vi "Update Slot Display.vi"(8 "error in":errorcluster, 9 "Location":cluster{"X":i32, "Y":i32}, 10 "Button":i32, 11 "UI Actor in":refnum<class "UI Actor.lvclass">) -> (0 "error out":errorcluster, 3 "UI Actor out":refnum<class "UI Actor.lvclass">)   [LabVIEW 2024, in "UI Actor.lvlib" / "UI Actor.lvclass"]
uses:
  UI Actor.lvclass
  UI Actor.lvclass/UI Actor.ctl
  Controls/Communication Parameters.ctl
  <vilib>/JDP Science/JSONtext/Next JSON Value.vi
  <vilib>/JDP Science/JSONtext/String Subset.vi
  <vilib>/JDP Science/JSONtext/Parsing/Advance past next JSON Value (inlined COPY).vi
  <vilib>/JDP Science/JSONtext/Parsing/Advance past whitespace.vi
  <vilib>/JDP Science/JSONtext/Parsing/Advance past String.vi
  <vilib>/JDP Science/JSONtext/Parsing/Advance past Number.vi
  <vilib>/JDP Science/JSONtext/Parsing/Advance past Line Ending.vi
  PDO Grid/PDO Grid.lvclass
  D:/git/Sourcegrid-LabVIEW/source/Grid/SourceGrid.lvclass
  <vilib>/JDP Science/JSONtext/Parsing/Parse Full Path or Item Name.vi
  <vilib>/JDP Science/JSONtext/Parsing/Advance past Array.vi
  <vilib>/JDP Science/JSONtext/Parsing/Advance past Object.vi
  <vilib>/JDP Science/JSONtext/support/Error Cluster From Code.vi
  <vilib>/JDP Science/JSONtext/Offset/Find Item Locations by Path.vi
  Sourcegrid-LabVIEW/source/Cells/Cell/Cell.lvclass
  Sourcegrid-LabVIEW/source/Grid/SourceGrid.lvclass
  <vilib>/JDP Science/JSONtext/JSONtext.lvlib
panel:
  out "Transmission Type":u8(ring)=254 items=["synchronous (acyclic)"=0, "synchronous (cyclic every sync)"=1, "synchronous (cyclic every 2nd SYNC)"=2, "synchronous (cyclic every 3rd SYNC)"=3, "synchronous (cyclic every 4th SYNC)"=4, "synchronous (cyclic every 240th SYNC)"=240, "reserved"=241, "reserved"=251, "RTR-only (synchronous)"=252, "RTR-only (event-driven)"=253, "event-driven (manufacturer-specific)"=254, "event-driven (device profile and application profile specific)"=255]
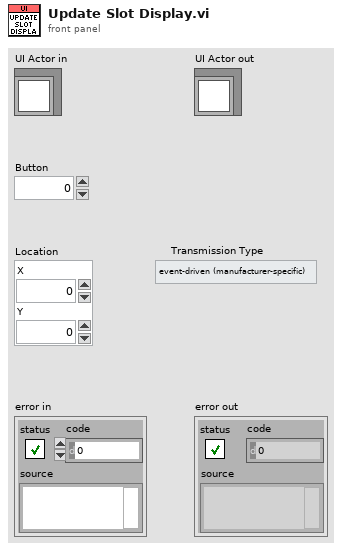
[diagram p1: front panel]
types:
  T1 = typedef "Communication Parameters.ctl" = cluster{"Communication":string, "Mapping":string, "COB":string, "Type":string, "Inhibit":string, "Event Timer":string, "Sync Start":string}
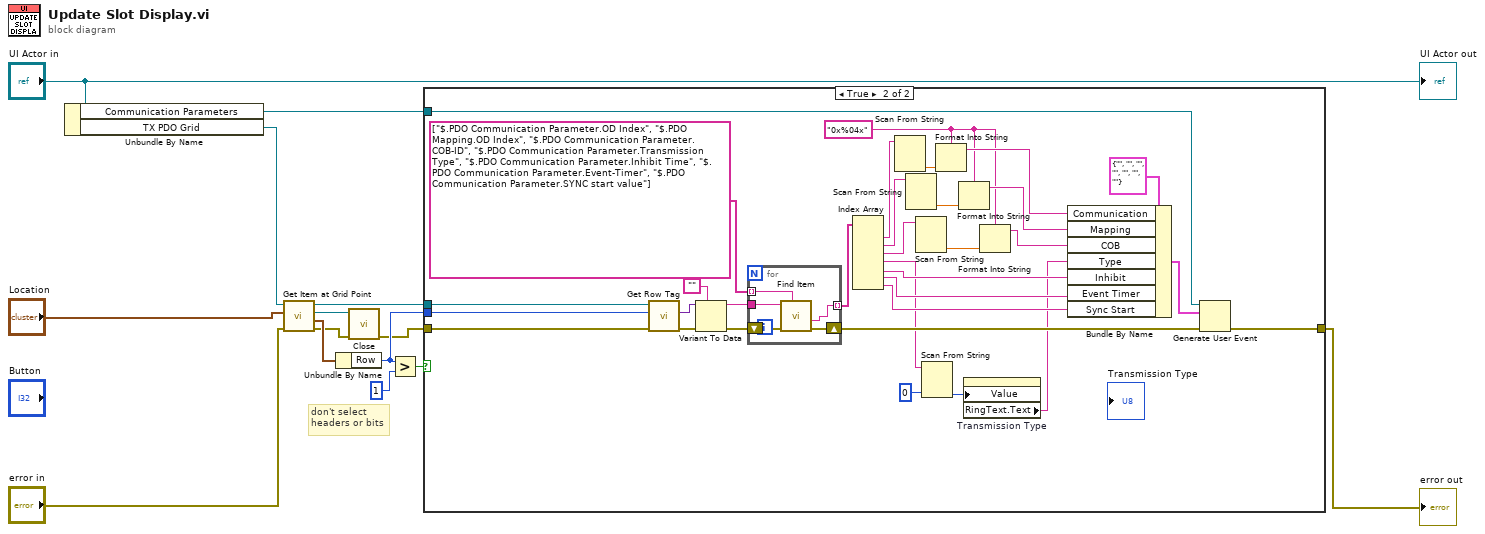
[diagram p0: block diagram]
diagram:
  # "don't select\nheaders or bits"
  n1 = Unbundle By Name("UI Actor in") -> ("Communication Parameters"=w1:refnum<user-event>, "TX PDO Grid"=w13:refnum<class "PDO Grid.lvclass">)
  n2 = call "Get Item at Grid Point.vi"("error in"="error in", "Location"="Location", "SourceGrid in"=w13) -> ("error out"=w8:errorcluster, "Cell Position"=w10:cluster{"Row":i32, "Column":i32}, "Cell out"=w2:refnum<class "Cell.lvclass">, "SourceGrid out"=w7:refnum<class "PDO Grid.lvclass">)  [unwired: 5 in]
  n3 = Unbundle By Name(w10) -> ("Row"=w5:i32)
  n4 = call-dynamic "Close.vi"("error in"=w8, "Cell in"=w2) -> ("error out"=w3:errorcluster)  [unwired: 8 in, 1 out]
  n5 = Greater?(x=w5, y=1) -> (0:w4:bool)
  n6 = case shown="True" w4 {
    tunnel: w3 -> [w15 w47]
    tunnel: w7 -> [_ w46]
    tunnel: [w15 w37] -> w6
    tunnel: w5 -> [_ w44]
    tunnel: w1 -> [_ w36]
    frame False {
    }
    frame True {
      w27 = "0x%04x" ("format string")
      n7 = call "Get Row Tag.vi"("error in"=w47, "Row Index"=w44, "SourceGrid in"=w46) -> ("error out"=w45:errorcluster, "object"=w43:variant)  [unwired: 6 in, 1 out]
      n8 = Variant To Data(error in=w45, type="", Variant=w43) -> (data=w41:string, error out=w39:errorcluster)
      n9 = for {
        tunnel: w41 -> [w49]
        tunnel: string[] ["$.PDO Communication Parameter.OD Index", "$.PDO Mapping.OD Index", "$.PDO Communication Parameter.COB-ID", "$.PDO Communication Parameter.Transmission Type", "$.PDO Communication Parameter.Inhibit Time", "$.PDO Communication Parameter.Event-Timer", "$.PDO Communication Parameter.SYNC start value"] -> [w52] mode=indexing
        shift-right: [w50] -> w38
        shift-left: w39 -> [w51]
        tunnel: [w48] -> w33 mode=indexing
        n10 = call <vilib>:"Find Item.vi"("$Path or Item Name"=w52, "error in (no error)"=w51, "JSON"=w49) -> ("error out"=w50:errorcluster, "<JSON>"=w48:string)  [unwired: 5 in, 2 out]
      }
      n11 = Index Array(array=w33) -> (element #1=w21:string, element #2=w18:string, element #3=w16:string, element #4=w22:string, element #5=w32:string, element #6=w31:string, element #7=w30:string)  [unwired: 7 in]
      n12 = Scan From String(input string=w21) -> (output 1=w20:dbl)  [unwired: 4 in, 3 out]
      n13 = Scan From String(input string=w18) -> (output 1=w19:dbl)  [unwired: 4 in, 3 out]
      n14 = Scan From String(input string=w16) -> (output 1=w17:dbl)  [unwired: 4 in, 3 out]
      n15 = Scan From String(input string=w22, default 1=0) -> (output 1=w24:i32)  [unwired: 3 in, 3 out]
      n16 = Format Into String(format string=w27, w20) -> (resulting string=w29:string)  [unwired: 2 in, 1 out]
      n17 = Format Into String(format string=w27, w19) -> (resulting string=w28:string)  [unwired: 2 in, 1 out]
      n18 = property on="Transmission Type" class="Ring (strict)"("Value"=w24) -> ("RingText.Text"=w23:string)  [unwired: 2 in, 2 out]
      n19 = Format Into String(format string=w27, w17) -> (resulting string=w26:string)  [unwired: 2 in, 1 out]
      n20 = Bundle By Name(cluster=T1 {"Communication"="", "Mapping"="", "COB"="", "Type"="", "Inhibit"="", "Event Timer"="", "Sync Start"=""} ("event data"), "Communication"=w29, "Mapping"=w28, "COB"=w26, "Type"=w23, "Inhibit"=w32, "Event Timer"=w31, "Sync Start"=w30) -> (w34:T1)
      n21 = Generate User Event(user event=w36, event data cluster=w34, error in=w38) -> (error out=w37:errorcluster)  [unwired: 1 in, 1 out]
    }
  }
  "error out" <- w6
  "UI Actor out" <- "UI Actor in"
